vi "Puzzle 25-1.vi"() -> ()   [LabVIEW 2022 SP3]
uses:
  <vilib>/Utility/miscctls.llb/LVMapReplaceAction.ctl
  832f64d6-6221-4642-9731-2bf24a069344.vi
  <vilib>/Utility/error.llb/Trim Whitespace One-Sided.vi
  c09a35fd-dfb7-4751-8a6c-d1f927b46256.vi
  c23b235e-6b21-46d7-9deb-4925a2cb368b.vi
panel:
  in  "delimited string":string="srp: gkb zst\ngrc: pxt\nrbc: zcc mth dgq zrv\nglc: dqz zlz hqm fkn\nzpx: sfx msc hnx vjs\nmlx: tpx mfb\nfds: zqn xcf brs nmv\nfjm: qdk\nrvb: kbj\nzcj: bmc brs jtm trk\nnps: bfh ths zds\nscs: kbj dqz zfb rtp\nqrj: jsk llj\nkdj: frn tzp qrj\nrxp: mkg\nqzr: cxn hnn vhf tdd\ntkb: bvf fhp vjt\nnjz: hlq fdc\ncmj: dfp\nhmr: vbd\nnnk: bnr\nfgx: lfq gkv kms mbx\nlqr: vpc hmr dsb\nsck: kbj skd\nqhk: hgs\nncs: bnr kxr ggq mdp\nqmb: bsf zqk fhq bsz\ntjc: bsq jgq\nzzz: jtl\ntgl: fvr sbc dqz\ntht: ptz qmp qmr\nvxl: mqs tkk bfc jls mzq qpm xzr ffx\nttk: qrx\nmxz: gtz\nhrk: crj scs xbm lqj\nbcd: gdl vtg\nnrf: mqf ndq fch zvp\njss: sks zdr phr zpt\nxhd: dpc\nfkn: hhl\nkgc: gnn\ngtt: bfc jrp jdd kjp\nngh: tlh chd tkz\nfzk: gdl hhj cxk\ngtf: mmt\npgf: nzk\npxl: jdx vqx vvq\nsrc: vcn cvg xjn\nzjb: hmv rfs thn\nnfb: qzc\nsbx: txq cms kcg\nkbx: jrc bnz lpg glg\ndjg: zzz nhs vvq\nbzm: mgb frt hhf mvq\nszs: qgx khz\nkcq: bbt xkv\ntkn: frn\ncbm: mmj\nlzh: nkp nbz\njvx: cjh mhz\nnrb: kms gtf gbg trs\nhkl: kvc\nbtv: dck\nqph: vnz tbb pbh\nfdp: hhl qkx\ncmx: tjj pnh prx\ntxk: qdq vqr cjv jtv\ntxz: kqd vgr kxn\nhnz: cmj\nmsc: fdc vjr\nmgl: ljf\ntzk: srv dbg\nckg: dfd pkx\nzzx: fhq zsm cbv ndd\nvpr: lfq zcc zzr ffm\ntkk: jbk xpp hpp\ndxd: xjn rjl kpl zjg\nmkz: qfv kfq kvc\ndkb: fjm mfr zxs xtp krc\nkhz: qrx\nkhp: fgm gkb kml jkz\nsxn: tnd htx dph rxp\njdc: kmr\nkbr: zqq zgx\nchm: dcv xbj\npdr: qmp xxd zkx\nzbv: bfv dln qct\nqlj: xsm jsk rtm\nkjg: hkl pcd\ngpp: stn qxq qjh kbz\ndtk: zcm hqs fjz flj cvl zcl\nlqv: lzm\nlcx: kxd krz bnz\nlqq: qtq vks\nctp: jdc kbs svx jqq\nfpr: hls nmv\nltx: pbh vcb qgh frc blr\nmmx: qkx vpc cct\ntsp: xrc zsq\nxdt: nfs spz\nxlf: dsb qft xfh xns ngx\nrmx: xps xxn mpt prc\nnmq: gmx vxd gms src\nklf: vgj mln\nfjl: pbd hvg jvg\nvzd: jgq\nqvx: rsq\npvp: rvb hqs xxd\nchd: jlk hqm\ngpc: pgc jvb\nzdx: nmk bbt shz vdr lzq\nths: btv zdr\nrtn: qpm hbk rpt mpm\ntdt: jnq xpt\ntpd: xjb lqh\nrgf: zqj\ntzp: xhx qcm\nsjs: mdb ncp\nkrz: hlq\ncjv: rks\nvgk: bcb\ndtc: vfj zqn qbk gvn\nckh: mtf jzf\nlxq: pkx chm\ncvc: fnv zqc mrp msn\nqbk: qxq kbm\njlz: mmp chf szf pbq\nqdp: mgl npj jpm\nddm: ljt gkd bkf csg\ntdd: rsg\nrhb: brb vhm kpl\nzjg: dfp\nxbg: hkb mqf\nszd: mnz\nsbt: kzl csp jdx nhr qgk\nczq: lzg\nfmf: grv vld rjb mbk pjq\ncnm: sqp btr xrk zjb\nxdm: shz bsj skd\nsnl: lkl drt kqm qnl\nhpp: htt\nmtv: bdh jnf\nzbk: hnz rvm djg zxs\nbjp: vfj bjn bbg zns rxp\npgm: dnl clq gzt kkm\nksf: bvf qhk nzc zdh\ndbm: rnh rnm smq zcx hjn\njbd: nrb xdd qgd\npjk: ljq\nghv: nrb kqs txh gnf\ndxp: vrh rst rgg vbs\nnks: jnq jrj bmc dkc\nnqs: rsn dfm rgs vng\nkfz: ltx vck lqj zxd\ncjr: nhs mdj bkp dkj\nvcb: qmr\nqpv: kjj fbk ffh\ndcn: kbj gtz\npvd: vhf\ngrk: qrj fbz bjn\ngnl: jmk mkl\nzkj: jhh\nzxp: pmb\ngzs: ltb ffh szd\nkvt: nzk\nhrt: flj\nvmm: qnf rsn hqg nkm npb dnh\ndsv: tzk pbq vfk tcg mtn\nzxd: vhc xbj crv ngh\nbvc: mcs zms sqg fnq\nxhz: szs\nckp: zlz ttb npd\nkmr: zjk\ngcz: dkv bzb pvp rhr\npbq: btg glm khc\ncqx: vgr jzq\ntbj: ddg zlx mtk gbt\nxtx: tbc lmg qqg snf\nlsq: gkb srb\nzlj: xxz qtc hpp\nvcs: kqd dsb jbk\nnrj: mzq xlf\nffr: csg kfp tgb\nmxb: tgj\nvsg: vhz cgt qbb\nqhj: cvl sks zrt\npml: jzq zfb fmg\ndlz: fzt\nmhr: cpx svx rkx dgd\nvhj: bns ptj\ndmj: fns vkl dgr\nvvk: mnz\njjb: hmg zsq qrj\ncxk: xln\ncvg: qdk\nrqn: nxm kkm\nzpb: cvg\nxjc: ttk\ngrh: gtx\nnnj: pxb vdp jdc srd\nghf: tbb dhd kxb\nqxq: rxs\ndpn: dvh ffr znv gbd\nmnf: thd\ndzz: spm ztq vjt\ncgk: dph nbz\nrhg: zpt\nnqv: gcp pzq cmj zvt rfx\nkrq: xrc rtm\nvtg: llq lts\nnkm: kvt hck\ngzt: ngh qdq\nskn: zqn spm gpc\nfnv: hkb\nbvb: dtm dqh hhf rsm\ntxq: pkl jbb\nfrx: kkm hxb ltn\nvcm: fzk rqn jhb bsj\njtm: bql mxf lkb xtl lcj\nnnn: csm prx khj qrs rck\nqng: gzq pbh\nvhl: smt\nxxj: rlj fql mhz kms\nzxt: npk pkm zpq cgz\nhtv: htn mvf xvd qtx\nntn: qbz zjg dlg qsl\nbjz: lxt vgj ncb\ncdl: jfc\nzvt: gnl sqp\nqgk: kfp jsp\njnb: bdh bjz hxb\nrtr: dbg jhs\ntcz: tvt\nbkf: ssk qhf lkn prx\nzlc: dlz zpb bsq sqg\ngkx: rcj dck vhh xjc\nrcj: tkz\nbmc: gnn\npsg: nmt dxk jsp mcj\nqqg: zst\nvng: cqx\nrxd: dpc hpp\ntcg: vhh\njnq: pzd tmv\njxx: pxg\nxld: xns fmg fdk\nqgv: kqd zlz mfh xdm\ntct: hck gzq\nhcm: hmv rst hsr\ncsg: hkp\nvln: msq frj vcs lhx ffj\nqqv: pmp khz\nbgs: dfs gmz jdd bsj\nngd: kdh pkm tzp\nfxr: zlv zbv nhr jrj klc\nhkg: pkl qrx ktl gjs\njdh: rfh hcm qkd ghb\njfm: btv\ngjt: tss hcd zgf hdg\njzx: hck kjp xrd bxs\ntlm: smt vhf\nltn: zfq mfq\ntbc: pcq\nsrz: qhq sbc xln mvp qpm\nsdf: mrn tpx mgl gbg hcm fqk\nfxn: msc vrh bfs vvk hkp\nqfx: tbc fvx jst\nrbr: cmm zxp\nfmg: nkk kgd\ngsg: bpm lnz\nsxl: crs\nznm: qqg rfv vms qrn\nghr: htt dcv\nzrg: gbx rdr tkz\nbnd: xcm hdg fds hnz\njbk: zpr htg\nbdv: nbz ptj vlk\nlvk: htt pcd\nhmn: qzs tfc csh qbz\nqhf: scf rgg\ndzq: qls\npjq: jbl ltq gcg\nsxf: vvq tfc\nthz: mrd bgm tfq rrc thg\nbsz: brb fnr\nxhx: tdk qlr\nkdn: pld bft fqk\ntcq: lkn mgb zgz\nsfj: vlh gft lxd\nfvr: hhl\npvk: tkm bbg tqb\nmdp: lrp hdg tgb\nqkj: nzk bmj nps xhq pgf\nmxf: zkj qcm zqx\nvlx: tvt cjv zfx sct\nxhj: jsp jtz hsr rgt\nlkb: bjq vnd fjl\nlqg: xtp zqn hjn\npms: xxz hnn htr gbx\nszj: zlj fjz xzr djq chz dmj jnf\ncxs: hsr xtl\nglm: nxm jhb pcs hrt\nqjn: trb pxk\nxnx: kgd\nmfh: svq lpk\nphx: scf\nzdr: gtz\nzzl: lvv ngd jrk qhk\ncpz: bnr szd zfz dzd\ntvr: vhj nhz pxk qtz\nvhz: svq kbg gkb\nbfs: cgk nnc gcp\nfqg: ffh\nkbm: pkm\njdt: zdh dgq\nddr: npx\nkmt: hdg hls gkr vzd\nxlq: hkk tqv zjt zzf\nxxn: mmx lbt xlq\njmx: vfg qsl zqj\ngvn: bvf dzq ccx\nkzv: mpk pnv\nkht: ddg\nlxh: ddk vjs mcf gzs\ntqx: ljq kgp\nvnr: sks\nqbb: blr nkk xfp\njmz: lkq dmx dfd bhv\ndft: fcg\ndpc: hhb\nsqv: nxc\ndjl: thd rrc\nmkj: vtk tlm ggr\nvxh: kxd ghq\nkns: zcx mxv gkc lzh\nvnt: dvj\nqrp: mtf pzr\npfs: mnf cfz sbx jfm\ntlp: xrc qzs tpk psc\nkks: mzl dsf ght svl\npxq: kmt jrj sxp\nvgc: shz ddr lkq rhd\nmrn: qdk\nqls: rfs tzt\nktb: llj mzl xnv lfz\nftn: dsb\nvrs: xpt fnx mzl jxv\nzxs: rtv rdb bvg\nbsf: vht\nlrp: zpb\ngpb: ngx jnf dnl gkb\nlcg: thd vnr tht\nmgt: dbg pfp\npvv: pqb znm spz gbx rsq\npdx: dgr qng srv\ndbc: ffx xkv\nbsx: src gnn\nzhp: nnz msq gft prc\ntst: rsg rgs\nlqh: jvb\npff: lxg lbf\njqh: frx flj ftn lns mrx\nxbm: prj tsb qnf\nthd: qhq\nvck: ztv vkl dkk vdr\nmxv: kxd tpd\nvcz: mtv lnh kxz nrf\njbb: pfp\nsct: ksj xbj vhc\nlkn: tkq\nfgl: ght snj xlh\npqb: vpp tvb vgk\nbgk: ptl zfz hls mdj cfg\ntxv: pld\nltq: qhf\nfts: mfr pnx cht fhq\npgl: rrj cdd llc mtl\nzdn: hsr bsm tsp bdv vxh\nsdc: zjg csh bjn\njph: zqc xhd jnc hxb fgm\nknf: qrn ndq lxt zpt\nnfz: jgr qgh bcb\nnnz: zkx fdk hhl\njtv: xhz hhj dfs\nzsm: bnr\nbpm: vdt\npcd: vng\nvgj: nvq kht\nfck: xjc\nxsm: fjm tpd jhh\njhs: hmr\nhtn: znv jch xdd hlq zsm\nsrm: nvf tnd cfg\njqq: cbm slg\nrsg: dsb\nvqx: sqv kgc tdk zjg\nqgd: lcx mdp ssk bbg\nmgb: mlq\nxpt: hcd lrp\nkxb: zgx vtl hch\nbsm: fdc kqt\nlzq: ncf pph cxn mqf\ntsb: vhf mxz\ntrs: qsl jhh pcr\nrzf: cct vhh\nhtc: fxd llb vgs mdb\ncrt: glg tvk fhq pxt\ngvk: csp sqv rhf\npqx: qgx jmv qzk\nzqk: tzt lfs\nzhd: qkd fxh mhz\nbrb: ccx\nmth: mxg lhb cmj\ntrq: sbl frn bns\nmvp: lnz zvp\nvmb: npd\nqmr: fgm\nvzl: llc kbs fqg gnl\nzfb: nfs lxd\ndln: xdd pzr vnd\njms: xjb ccx mdj lqg pnv xjn\nvhc: kjg kcq\nffj: qvz\nqgh: lqv mfq\njcv: lfs pff zqx\ncxt: qhv cvd svl kpl\nzxc: qqv fxq djq htt dbc\nvjr: spm ghq tkn\nmht: zqx qtz xrk glk\nsgx: chm bcd rzf mhb mnf\npxp: jmk\nvld: jbx rst zns vnc\nkcd: dgr\nmlj: hnz hns rxj\nbbm: hkl lhx mqs\nnvs: rqn gtt vlh fns\ncqh: gzq\nkxt: pxb jdk gkr sxp dkc\nhbm: vxm bfh\ntgb: pbd\nhdl: kjj dmd mmj tdk jtq\njcq: vfg rtm tmf glg xjb\nqkd: dsf vxd\nnzc: grh fgl\ncpg: mmj mcf tlp\nlns: vfr slb htt cdl\nlps: cxk frx fvr msq\nfvx: fxz htr\nffn: psx bcb rhd jvz ftn phr npd\nstb: djg trs sxl lqh\nkmj: rtm pxt rhf\nqsn: vbp qxl fdc\nsrf: kgm rvm fbr thn bsx\nmdb: slb blt ddr\nggr: qnf\nlsh: jhs rvg gmz\nqfb: lkl qfq dvj\nzlz: smt\nzfx: jvq qqg xcq\nrmd: phn gfn frj\npsd: qnh vmb nrj qnf\nhml: mxt\ndbx: lvk kxn xhd vbd\nncf: kqd mtk qrd rgs\ncbv: sdc\nbph: pxl fdf jpm lpg xhx\nfmr: kxh hrg prj\nrhr: kmg kng gfn xcq xlf\nslg: qxl dqm nhz tgj rck\ngdh: znl vsr qnf\ncbn: zfq vms mrg rfv\nblr: hkk xfh\nmcs: cmm jtl nzc xgh\nmmj: lqh\ntvv: ltn cqh srp rtr\nzfz: krb\nshz: jbb ztd fch\nght: qbz csm\ndcv: nvt\nzzf: jst jdd kjp\nzmx: msn rzf rhg kcg cfz\nngz: xtz qhj lnh vgr\nxxx: vgs tvb\ncjh: zns\nsbl: dxp kmj\nrjl: tgj\ndjj: ktq ttk xxx\nqzd: fgg\nklk: jdd vgj\njrb: sqp pxq nck rkr\nzcm: mln cqx mdd\nbkk: tst rrc mmp\ngkv: mfk ssk csg\nthx: ftn sdm grl fdr\nqmm: qfb hbg qsn\nkml: bqd\nbfz: srm vht btp\nfsx: bkk zpr jmv mzq mst hxb\nncp: rhg\nncq: qfb dmd tgg\nrfx: bbg jqq\nzgz: krz gcg ghq\nthj: hmg sqg zjg mnz\nxxd: sks spz\ndxm: ndd\ncgt: vmb llb trg\nrql: mkl pxp cgk rkr\njzf: qrp pxb\ntkm: grf\npmp: qtq jfc\nvnb: frd nfb prc\nszf: frc mln qhg plt\ntfq: dgr hkb\nvks: ztd zlz gbt\nzsv: lzh tkm hgs\nkqt: tch njz nnk\nnpd: zvp\nfpx: hnn hzg qvg\nzzr: jvg gvk cgz\nsnn: bnz pkt djg mfb\nlxg: fhp\nxfp: kht\nvqr: qtc jhs szt\ntnh: ngq hjn ljt fsg\ncms: ffj kjg\nqrd: cvl\nrjr: btr cjh rlj sqv\nsfq: jdx fqg sqp ngd\nczj: sdf psg tkq qhv\ndbq: pkl vlp snf trg\nrjb: xhn sqg\nkhn: gvq gft\npxg: fqg pld\nhhb: npx\nkgm: kfp dxm\nqfv: qmp pgf\nmsb: xqq jfc dsb fvt\nmrd: vxm\nmdd: kjp\nxfg: gvq ggr zpr nkk skd mrp\nrrm: bkp vxh pvl vlk\nvfj: mbh\ngbg: cjr czq\ntkz: frj\nqfr: rfx hnz rdp nrb\ntqv: nsh gzq rdr\ngrv: lzg\nzgf: dlg hzb qlj zpq hgs\nngm: gxf szs kcq hzg\nqln: lqr jsm hmr gbl\nzcl: bcb rrc jzz\nvlt: kgd mtl\ntch: mmj rjl kjh krz qhv\nqdg: kqd lxt vxm qvz\njnx: lxd thd pdx bcd\ncrv: ggr sxb sqr\nhsr: tmf zjk\nfmj: scg dft lxg rxp\nnpb: kcq msq tsv\nsdm: mrd\ndfp: mmt gtx\nktl: jth gdl slb skx\nddb: trk csp mgl lzj\njzr: ckh dph brs kmr\nmnt: srp xtf gqz\nzqc: xvf srb\ntpk: rdb\ntmn: kbg kjg jxk chd\npnh: qjn tpx lpg\njnf: kbg ttb\nthg: mxt zjt vsr\ndnh: xft gbt\ndbg: flj\nzbn: hlq tlp zhd xjn\nbzb: qdq dpc\nmmp: mkk vhl\nmbm: znl\ntxh: dvj\nfpd: jbx zxp qpv\nrdt: ptl jrk fzx\ngpj: mrn\nrzj: kbg tsv lpk\nvhh: vpc jth\nsqg: tpd mcj\nhlf: dck tcg sck fsv jss lfr\nzcx: mxg xkn jsk\nxnv: xcm xkn\nnvq: ktq\nrzz: lvh sqp dtm hbg\nprx: xjb\nsxg: rbr sxl pbd\nvlp: gfx gft\nltc: bql pzr gvn\nhck: htg\nqtk: nbb mbm mkk\nksj: tvt\njbn: qzd ffh lkl\nnhv: fql kdn\ndzk: hqm lsq xbj rxd fnv\nkgn: gfq ltb pvk jbx zlf\nlsv: qrc rtp kxz chm tlh\njsm: hcj bzb mbm\ntbb: bbm nvq\ntgq: cmm vnt grf xpt\ncvv: mvf xnv gnl ngn\njmn: tdk rzn rxs cbv\nhbk: fxz\ndkv: srb mdd slb\nzlf: dvj\nnkj: sbl svr pxb krb\npgc: kmj\nrqg: grl nlj hzr tsv vhl hhj\ndkk: gqz qft vlh\nzzs: hjp bvm pgc ggq vvk\nqfm: tfc tsp smq mfb\nmvq: gfq mlq\nfrd: fch dfk\npsx: mrg djl dmx prj\nbvg: gtf tzt kxd mxb\nbfc: phn\nfxx: hgs qbt knc qrp\ndqm: vxd zsr\njhm: zdr gbr ckp fkn nrj kgq\nxjq: htx khj\nchz: nxm svq szt\nsjt: pnv\nvfg: vht kzk hls\npqd: gjs vdt zlx blt\nrcs: pnx hnt jpd qff\nsvr: tgj\nvqc: qfq\nnbb: bdh ncb\nktv: trb vzd\npph: pbh cct\nlkd: lbt lsh zcm xxd\njrp: njh dcn qhq\njbx: rjb\nmpm: qnh ncp qrd pml\nbsq: qbp\nbdp: vzd kxr bhj mtf kjh\nqft: ztv\nfxz: xpj qrx\nfrn: dxm\njrt: xrk bsz rfh\nrhd: xpp jlr mxq\nfvb: gtx rkb tcq hbx\ndrt: gkc mhf\nfnq: jnq xlh vsm lvh\nffl: khj\njvb: qxl\ntlf: rrc dfk gxf bcb\nvbg: tlm hhb vpc fmr\nmbh: cmm\ntgg: dvh\ntgx: qhk mvq fcg dxd cvg\nrtp: jvq cxn\nzxb: zkv tvb vdt gbx zkx\nvtl: llq qzk rcj\nvdc: xrb\nbbs: rjl\nxsg: jnq gkr mdj jzf\nkqs: nck qkl vss sxl\nzdh: dsf\njlm: lzj mcf qcm zkh\nzkn: xkv xfp qzc klk\nkmg: rvg kcq\nfxc: rdp cnr zxs kzk jch rgg scf vcn\njxc: spf hbk\nbgb: nmt qrs cmm svr\nnlj: hzg ncb\nngn: rfs crs\nbjx: ztd kvc\nrkn: fqg bzc kbm dmd\njsk: tjc\nktq: chf\nxrk: tkb\nlld: lqv mnf\ndnq: hvt krb cpx lkn qnz\nttn: qnl cxs tdt llj sxl\npng: sdm ghr mtk\nhjn: bsq\nsmq: qcm ngn\nvnc: bsf dgq shm\nlfq: dqm qbz\nvgs: gqz\nxnf: hdg kjj mfk jdc\nzms: crt fbf qdp tmv\npvn: mfk svx zns htx fbz\nnkf: rsn fck gpb pcd\nksn: csh bfv phx\nvhm: mqv dxm bql\ntfc: mxg hzb\ntnp: ffj lld\nrhf: qfq\ntxj: srb vsr btg rvb fns\nkzp: jrt qhv nzx tqx\nngq: pzq bnr mht\nnbf: cbv sxp jrc hjp\nkhq: sqf pgl rtv dxm\nmtq: zqx kbz frt nck\njzq: frj\njhb: xpj qtc vhl\ngqx: mqs zfq qnk\njkx: bfz pvl gkd frn\nqnz: vxd qzs\nhns: qzs zlf\nzds: qkx xfp\nhjp: jrh nnc\nqst: qzk kbb mnt smn\nvfk: sqr xqh qzr\nvpp: xld hkk kcd hkb\nmkl: zqn\nbpk: hzk llq xns kht\nmvf: pxg\nkbz: zlf cfg stn\nxgc: gcp jzf vbp gmx\njks: ztd znl rfv\nxdq: mlj ksn nxc ljf kqm pvl\nmcf: frn\ngbb: sbt fzx zsr plf\nlfs: jnq kdx\njhc: llc vvl mbh qkd\nptl: pxz csm\njtq: ddx\ngzv: cms ncp cxn\nprj: bfh\nrrc: jzq\nkxr: rvh hzb csm\nvbv: vdc jkx rkx tkm\nxft: ttb\nddg: bdh\nxcm: jrh dlg\nhdc: jgq cxs bsx pzr\ndkh: zhd kdj jpm jvg\nggn: ttk cqh jth\npkt: zvc khj bhj\nnhs: ghq\nrdq: jzz vnr zrt\ncvd: llf kqm rck qfq\nzsc: jpd pmb nhv scj htn\ndgd: cxs bjq qpv\ngbd: bvm mxb jdt\nvdp: jgp dvn rzn\njkz: kfq npx\nzjt: qvg qrn\ndrd: rst hns jrk mrn\ndtg: bbj gkr rjh\nztq: jvb pxz nhz\nxln: gbr\ndgq: svl\nzfg: gtf mvf ddx sqp\nlkk: kxh pvd ljr gzt vnr\nmhf: ghq mlq\nhqr: scg rxj qkl tkq\nmgm: ptj pbd rxp rtv\nlzj: xcf lfz\njtz: jpm snj krb\nsfg: xng dvn fdm kbf\nqff: csp pxz\njxk: mkk qnh mbm\nxpj: jzz\npcs: ztv lnz\njrk: xkn rkx\ndzd: krq tfv xth\npsr: rlq fsv rks gzv\nfrc: nfs\ntjj: sfm\nzkh: bsq rxs\nfjz: srp\nkxz: cxn jqv\nscp: cpg tgq ptb qzd\nxtp: qbp\npns: hhb cdl\ndzj: cgz gpj lkn gkc\nfvc: rrc hqm ngc xjc\njhh: bvm\nplf: xgh sxg nhs\nllf: ffl xth hdg\nbjq: ddk gms\ncrj: ngm ngc vlt\nqhv: jtr\nvss: pmb pxn bjn tfc svr\njnt: fcg jxv tpk kbf\nlrh: chd kbr hqs ztv\nhzb: txh jrc\nrkx: nnk\nxns: kgq lhx\nkcn: kkm zrt lqj xbv\nxrb: mmt zsr mdj\ntqb: bds mkg kdx\nblt: lzm\nxbt: skn dzq kgm qlr\nrvh: shm jxv\ntrg: btv\nmrx: tsv mfq\nxtf: zpr vtk\nzqq: rzj vbd\nxrc: mpk brb\nbkj: pff zbv mgb crt jbn\njvg: fpr gnl scg\nlbf: xpt\nxzr: znl\npjn: trg qft pvd pgf xft\nccx: mhz ffh\nnvf: kms\nlkq: zqq\nbtg: lxt spz\nrlj: kmr kqm\njqg: mkz chg xkv ncj\nxth: vcn\nbhj: vht bsx\nxvd: ggq qgd trb\njgp: ltc tzt mkl khj\ncqt: gkd gpj qht krn\ngmx: qsl zxp\ngjs: ksj mtl\nqtc: qzc\nhvl: gcg gkr fnr nrb\nfxh: nkp svx\nrxj: pkv gfq\nfnx: lvh kgp\nmhb: mkj nsh qpm xqq\nchg: pfz rqr lqq qft rsn\nbtp: rgg vnt kgc dkc\nrzr: vrv nkj grk bds\njpd: vvl mgm\npkv: xth bbs rrj ggq\nkdh: gms gnl\ntpq: mvp qnh kxn\nkrc: mxg bnr ffl\nvnd: hmg\nzlv: mfr bft dzz\nnfg: jlr ksj nvq lnh\nrld: lxt svq hch\nspf: ptz nfb htc\nvdt: rhg sxd xtf\nhvt: trk rnh bnz\nlfr: qvg tst xft tcz\njtg: jbd lqg hcm rvm\ncdd: brs kdx npk\nhqg: gmz xhd frd\nbgm: qvz vnz\ngfn: bxs\ncrs: fql\nvcr: xcf pxn jsp shm\nvjs: lzg jtl\nlfz: kjj tjj\nfdq: pqz qbp qcm\nlnh: zfq\nnmk: kxn xtc phn\nnpj: lkl mlq mfk\ntcc: tss nhz szd kns qzs\nlts: jfc sbc\njbl: ndd\nkgd: jmv\nsnf: vms\nlmq: xxx bpm djl vng\nkbs: gpc\nphn: kgq xfh\nkzn: thz blt mxq sct hml\ndts: hvt bql ggq\nvvl: zzz ktv ksf ght\nllb: gqz\nvlk: jdc mnz\nljr: ggn vnr nvq\nfdk: bbt\nnkk: snf\nqbh: krz tdt cvd rhf\nhxq: jmx vdc dvh cbm\nrll: rdr mst jnf vgk sbc prj\nhzr: tbj jjm xqq\nzrv: lrp grh txh\nqtx: jcv stn tkn\nlph: rjh nmt crs kgp\nkxd: rhf\ntvk: pfd pjk\ndhz: gbr gfn fdp kbr\njrh: scf\nngc: gss hnn xnx\nzqn: rtm ktv\nqgx: nvt\ngrd: rrj bsz qjn lzh\npfz: ncf tnp qdq\ntzt: zkh\nzhh: thx mst tsb xhz\nxqh: tct bxs kml vmb xzr xbv\nxpp: xfh nzk\nlzm: mxz\nbtr: jtr krb\nzmt: jfm zxq fmg chf dgr\nmcj: nmt vcn vjt\nkcg: szt jbk\nqjh: pvl drt ktb\njls: tlf pns\nnbz: vjt\ngcg: txv fnx\ndfn: kkh rsq kmg jnb\ntss: nlh xmq kzv\nlbd: jmv gqt nkm ngm\nrfh: trk\npzq: svl hcd\nfdr: vsr blr ngx nlj\nljt: zsq tmf\nxlh: txh rhf\ntlh: nbb xjc\nfhh: fck qvz lcg ggr zrg mrg zrt\nhsp: vnd czq pbd lzg\nvsp: jhh fqk jtj bsm qff\nrnm: ffm jtq drd tgg\ncnn: mbh qnz kbm jrc\nptj: jdk\nxng: nhr jnt pnv\ndqh: mvq qgd dlz\nhbg: grh tjc nnk\nvbp: trk vbs\nrsm: glk ffh ljq\nlpc: vcz jgr lxq\nszt: mln lts\nnmf: ddx bvf zsv sxf\nnxm: gqt\ntcn: dbg gbt lmg dfk\ngqz: tvt bqd\nfbr: zsr fpr qct\ngrl: kgg ggn\njst: kht\nmxt: frj\njqv: mtv gtz jvq\nqhg: npx\ngdl: gsg\nvlg: jjm xsq tbj vgk\nsrd: vqc\nznv: fcg vcn\nhnn: kht ptz\nlpg: gmx pkm\nrdp: zvt tpd\nxtc: ftn kbb jlr zgx\ncfz: lqv pkx kml\nxtk: xdt lcb qpz txq pfp\nhhl: lpk\nbkh: bqd ckg rkv jkz\njlr: gss\npqz: pdq qhf jdt\nlrm: skx tsb hbm sfj bhv\nsbd: ncq fhq zsm pxn pxk\nxcq: xbv qpz\nvcx: htg bbt tlf gzq jfm\nnlr: ddg dfk ncf kcd\ndbn: dlz mqv qrj nhv\nzkv: hkp kzl\nnsh: rks pph\ndfs: jzz pns gss\ncgs: ssk zpq dtg rgt\ntdg: zdr qkx psr qtk\npfd: zqn mdj\nrvv: sqf xdd jtz snj\nrtv: czq llc\njvz: nzr qgx qfx fkn\nclq: bgm tpq bxs tdd\nfzt: hjn rfh\nmrg: sxd bjx klf\nfmx: pjk pxp svr rgf\nkbb: mdd sjs\nlqm: kvt rks qvx\ntfm: bjp mnz shm dxk\nnlh: rdb bmc\njjm: gfx mnx lqq\ncpx: pcr mmt\nzlx: dbg\nqnl: kbz sfx lcj\nccp: rrj jtr rvh tkm\npxb: bbs\nkvm: skd fgm txz\ncsb: mlx sfx cbm gcp\nrnr: zvp fvz kng vkl tcg qtq\nfbk: jxx xpt bnr\nfxq: pcs bjz vfr\nkdk: qtz jxv vvk\nnnc: rfs\nlbt: gqt hbk\nfsv: mrd cqx\ngqt: kgd\nvnz: hkl rsn\npcq: dsb khz qpz\nhgs: pzq kzl fgg\nkpl: tpk mkg qbp\nddk: ffl\ncbc: jsh lcj dxm tfv\nvfr: xsq txq\nxsq: ttb\nhch: kgq smt\nmhg: nfs bzb xsq tcz dcn\nhmv: rst jxv\nbbg: bbs txv xcf\nzvm: zcx kgc trq htx\nlcb: mvp frc kcd rxd\nnck: qzd bsf\nngx: mtv\nkvc: llb\ngfx: fch ncb\nzlr: sxf qrs psc kjh vqc\ndlg: rgf\nqzk: jlr\nbzc: tjj nvf hcd sjt\nhfp: sjt dxk qxl zpb\nlvv: fnr nnn bsf\nsqr: tct skx\nmtf: njz\nmst: xpj\nlcz: rrj jxx dft jqq\njgr: gvq hkl\nxrd: fvx zkx sxd lkf mfq vbd\nvsm: sfm bmc\nmrp: mtk ghr\ngfz: ths tzk jfc txk\njtj: rrj hnx cln\nxxt: hnx xdd rgt lfq\ngxf: cct\nsrv: cdl mqf\nfdm: ddk rxs pcr\nccf: rld lhx rdr xlq rtr\ncgv: hzk png vnb phn\nhnt: qrs fdq glg\ncht: ddk cmx\nqrr: mbx phx bft hjp\nhtg: fdk\nfbf: jbl hdg vvq\nqnk: ths bjz jls smn\ntqs: zqc rgs vlp lld xxn\nkxh: qgh bpm rkv\nmpk: mhf rgt\nzsd: stn pzd qdk sjt\nmtn: hbm vng\nhmg: kfp\ngmn: zds mfh gbt chf brc\nvgr: qgx\nblm: vgj ctb rtr lpc\nskr: vrh tfz rgf xtp\nphr: mrx nvt\nknc: nnc tlp bzc\nqlg: kgg zpj pqx lqm rfv\nqbt: jxx rhb qxq\nxnk: lhx hbk dcn xtf\njsh: grv gfq pfd\ncln: gpj zns vbp\nnjh: mst mxq\nmbk: qjn kdk ltb\ndjq: vtg dnh\nplt: snf lxq hbm\nncn: mkg tfz ztq\nbmj: lkq vtg rxd\nqsh: vsg qlg pdr xvf\ntvb: pvd\nqkx: tgl\nlqj: fns\nqtz: fjm grc nmv kqm jch\ncfg: dvh sfm\ndhd: sxd vdr rfv\nkgg: lxt\ndlh: fvr vlt vtk tcz\nzpj: lnz bbt xbg\ntnd: gnn\nlcj: tfz\njfn: rsq dfk jks rmd\nzxq: mtn lpk hml\nsft: npk zfz qsn jrh\nvff: dlz qct krq pxk jtl\nqpq: qng qmr rgv ncp\njlk: zgx qtq hzg\ndvn: grv xsm\nmsn: fck xxz\nrzn: zqk mxv\nplq: mxt sjs bqd dck jbb\ntzs: lxd mtk xsq rvb\nhzk: pkx\nthn: nvf pjk pdq psc jxv srd jvx\nnhr: tgg rck\nmtm: pfp qrd hhj fns\nskx: kjp\nfrt: fzx grc lzj\nmbx: csh kms\nhvg: qct srd qgk\nhnx: gkc dsf\nbds: bhj dzd\npzd: jmk csh\nndq: gxf xnx\nkfq: xjc\nrnh: zpq xjq\npkl: ztv\nprc: mqs\nsxb: gbr vcb ddr hkk\nrlq: gvq qvg\nnzx: kjh dxp jjb kbm\njvq: zst\nfss: zst nfz znl nsh\nhbx: vfj mlx gtx\nbns: xjb pld\nmfb: lbf\ngzk: qlr rdt fbz kdh\nrqr: zrt hrt xln\nmpt: vdr rlq smn lqv dbc\nbrs: src\nsqf: jvx pxt dkc ksn\nrjh: llj vqc ltq ghb\ngkd: lbf\nxmq: sjt ncn pxt\ntfv: bft dfp\nsfm: spm zjk\nghb: zqj\nxxz: pfp\nffx: lsq tlm\nfqk: jch\ncnr: pxn tnd scg\njnc: qhq qhg gfx cvl\nddx: dph\nnxc: fgg nkp\nzcc: vcr btr\nmxg: zjk\nlfp: rnh gpp bsf psg\nqtp: nvs bfc jxc zlx\nkqv: xjq jtq fxh txv\ntkq: zkv\nscj: zqk cjh cht\nmqv: phx pfd\nctb: fch lqr djj\nmfr: zxp vxd\nbsj: lzm htr\ndtm: mxb grf tkn\nfnr: grc pcr\nsfx: ljf fgg\nvbs: vqc tmf\nkrn: fhp vsm mlx\nxbv: qvx\nptb: vzf nlh pdq ljq\nkbf: dkj fhp\ngkr: rdb\nqrc: ckg msq qvx\nhqs: hck hzk fpx qmp\nqrn: vxm ktq\nkhc: pns ktq qmp\nlmg: lqv xtz\nkfn: shm qxq qkd xtl\npxn: mzl\nsfr: ndd zkj hbg qhv\nhtr: jdd\nvjl: kfq jph mxk khn\nbfh: jth\ngmz: xnx qpz\ngkk: jdk qhf ljf bvm vrh\nkld: bjx qzc kgg rkv\ndkc: bfv\nxlm: pdq tgb fzt zxp\nfvz: smn qhg fzk fjz cqh\nrpt: phr qmp mqs\nntm: tvk mlq rvm ltq pld\nrrj: sxp jgq hkp\nxps: qtq vhh ndq\nfdf: hmg pgc tpx kzk\nbbj: psg dft nkp\nkkh: mzq xqq rsg ksj bqd\ndfm: blm mxk sck pdr\nnzm: gcp pjq qbk zqx bfv\nmxk: mgt qph vcb\nptz: gdh\nffm: kdx\ndkj: rlj glk\nlrz: zlj znl zmt kvm\nvlh: zpt mln\nrvg: hch\nbkp: jdk kgp\nfzx: kzv\ndxk: nhz\nbnp: btv kbb tdd ghf\nmnx: vms gss vng\nghq: rtm\nfsg: svx dlz kbs\nfxd: mxz nvt klk dmx\ngrf: nmv\nklc: grf qkl zqj\nlkf: dmx scf vpc tht qqv\nzvc: ckh dzq jsh\nvnx: vzf jbl pzq kzl\nrkb: dts qlr lvh tqx kdx\nxgh: ggq pmb\nmkk: mqs\nvpv: zsq ght cjr qkl\ngnf: phx zzz xkn jtr\ntnr: gqx hml qfv vks\njdx: jrj mvf sqv\nccz: khn msb ksj lnh\nkzk: pzr\nxcj: cbv vhj bvb rkr\nrkr: npk\nljl: qsl glk trb vnt\ncxf: bjz nfb njh cjv vgs jxc\nhvs: fpd jsk mvq rhb\nvrv: dmd nnk qmb ffm qls qmm\nqzc: mtl\nxtl: pxz\ntfz: hhf jgq\nxvf: vbd tkz\nfbz: vvq\ngms: fql\nxhq: qtp nlr xbg nrf\nbhv: gsg xns\nnvc: hlf qph mrm sct\njmk: hhf\nvzf: snj pxp\nvkl: mgt rdq\nbrc: pmp sbc mxq\npnx: mgl hnz\ncgz: qsl\ndnl: jst dcv hch\nxhn: ltb svl hdg\nncj: tkk kvt lvk\nhzj: vdc ddx vnd pzd\nhcj: dqz rkv cxk\nqht: lxg psc kbf\ndfd: thd lpk\nkng: chg tbc\nhrg: xtz btv hrt vgs\nnzr: zgx xtz vtk\ntmv: rbr fqg pzd\nlhb: ghb lzg zkj zdh qbz\nfvt: klk sdm tnp fdp\ngbl: xhz fnv rvg\nrgv: fxz tfq bsj fpx\nmrm: llq klf qvx xdt\nsrb: rcj"
  out "Set 2":set{string}(c389)
  out "nodes":set{string}(c389)
  out "Map":map{string, set{string}}(c390)
  out "String":string
  out "Set":set{set{string}}(c389)
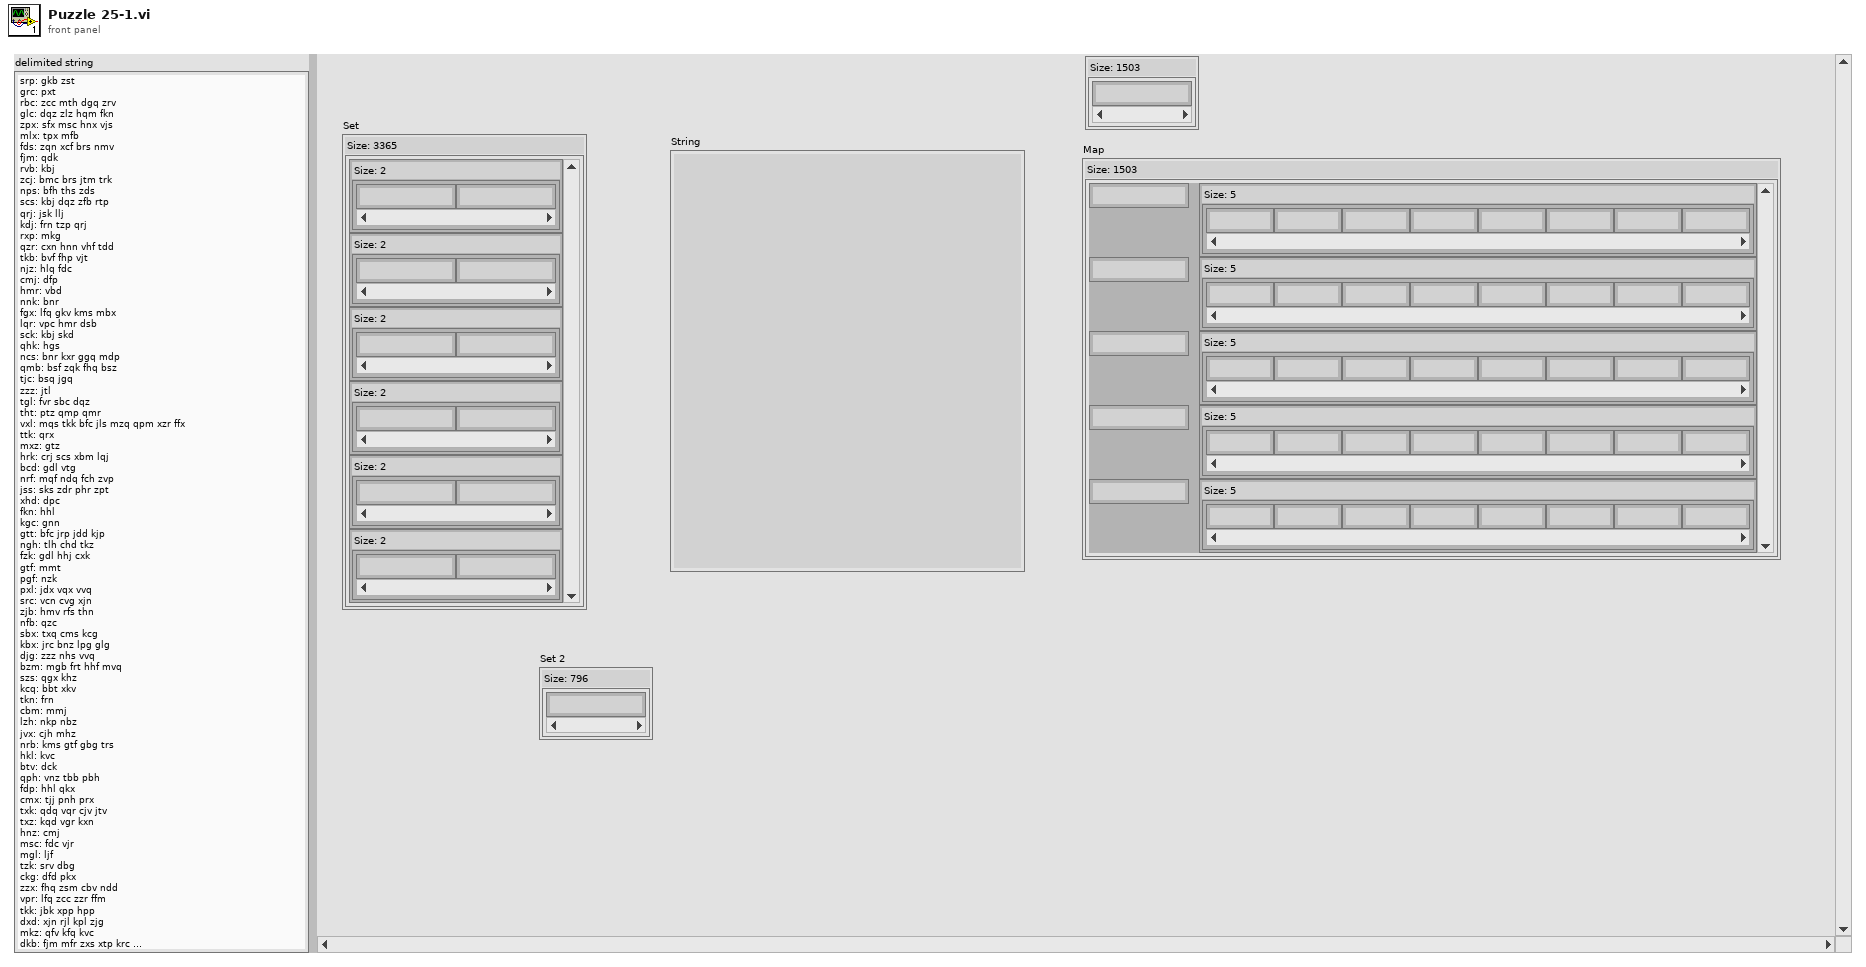
[diagram p1: front panel]
types:
  T1 = typedef "LVMapReplaceAction.ctl" = enum32{"Modify Entry only if found", "Add or Modify Entry", "Delete Entry"}
  T2 = enum16{"open", "replace", "create", "open or create", "replace or create", "replace or create with confirmation"}
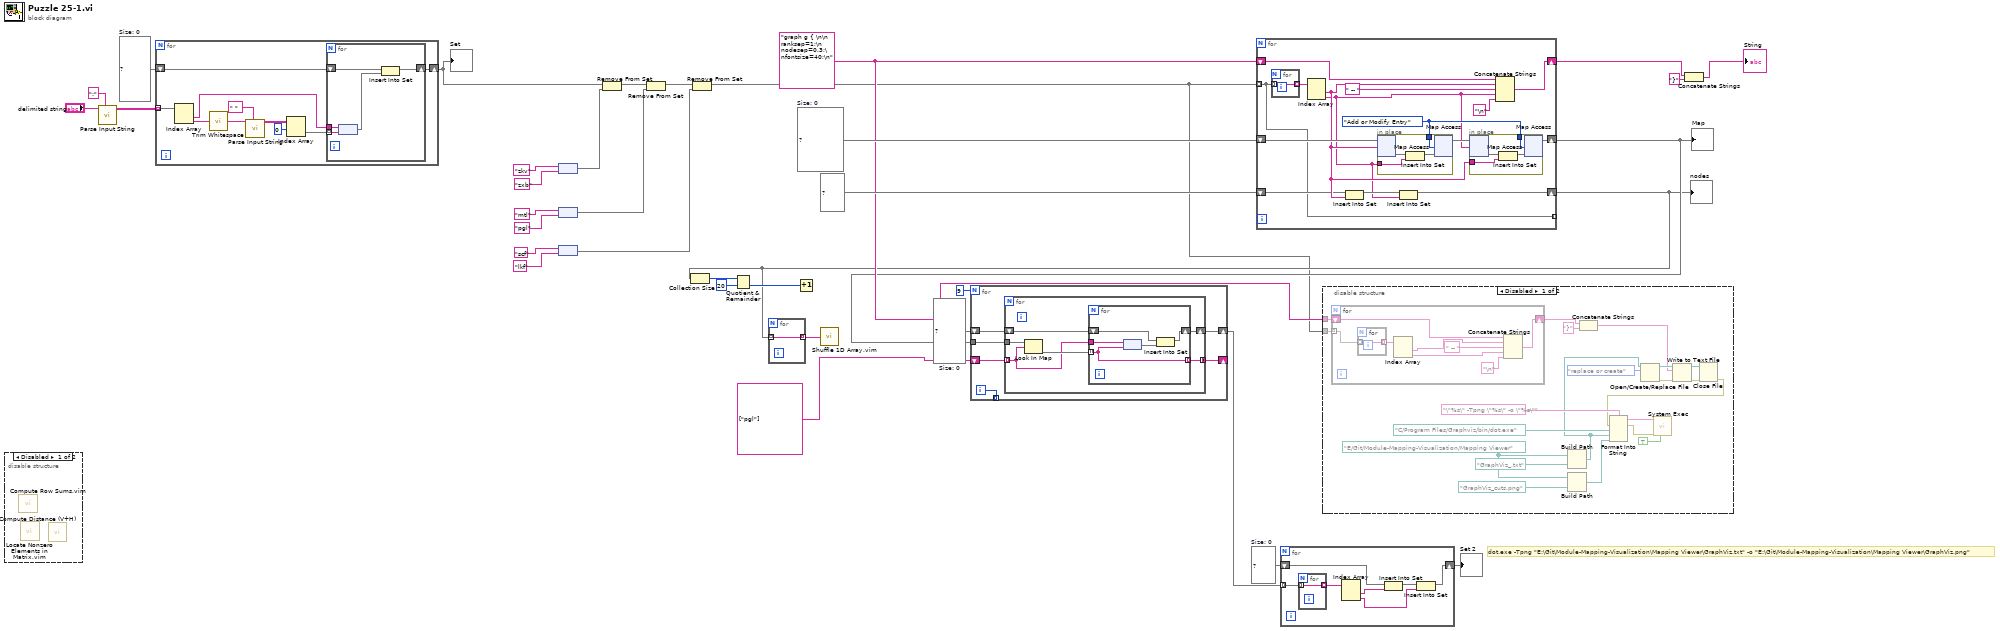
[diagram p0: block diagram]
diagram:
  w2 = set{string} {}  # Size: 0
  w18 = set{set{string}} {}  # Size: 0
  w24 = "graph g { \n\n    ranksep=1;\n    nodesep=0.3;\nfontsize=40;\n"
  w31 = map{string, set{string}} {}  # Size: 0
  w32 = set{set{string}} {}  # Size: 0
  # "dot.exe -Tpng \"E:\\Git\\Module-Mapping-Visualization\\Mapping Viewer\\GraphViz.txt\" -o \"E:\\Git\\Module-Mapping-Visualization\\Mapping Viewer\\GraphViz.png\""
  n1 = disable-structure shown="Disabled" {
    frame Disabled {
      n2 = call "Compute Row Sums.vim"() -> ()  [unwired: 11 in, 1 out]
      n3 = call "Locate Nonzero Elements in Matrix.vim"() -> ()  [unwired: 11 in, 1 out]
      n4 = call "Compute Distance (V+H).vi"() -> ()  [unwired: 11 in, 1 out]
    }
    frame Enabled {
    }
  }
  n5 = call "Parse Input String.vi"("delimiter (Tab)"=":", "delimited string"="delimited string") -> ("parsed string"=w33:string[][])  [unwired: 9 in]
  n6 = for {
    tunnel: w33 -> [w45] mode=indexing
    shift-right: [w38] -> w16
    shift-left: w32 -> [w37]
    n7 = Index Array(array=w45) -> (element #1=w39:string, element #2=w44:string)  [unwired: 2 in]
    n8 = call <vilib>:"Trim Whitespace.vi"("string"=w44) -> ("trimmed string"=w36:string)  [unwired: 1 in]
    n9 = call "Parse Input String.vi"("delimiter (Tab)"=" ", "delimited string"=w36) -> ("parsed string"=w42:string[][])  [unwired: 9 in]
    n10 = Index Array(array=w42, index (row)=0) -> (element=w40:string[])  [unwired: 1 in]
    n11 = for {
      tunnel: w40 -> [w49] mode=indexing
      tunnel: w39 -> [w50]
      shift-right: [w47] -> w38
      shift-left: w37 -> [w46]
      n12 = node(w50, w49) -> (w48:set{string})
      n13 = Insert Into Set(10:w48, 11:w46) -> (3:w47:set{set{string}})  [unwired: 1 out]
    }
  }
  "Set" <- w16
  n14 = node("zkv" ("element"), "zxb" ("element")) -> (w4:set{string})
  n15 = node("mtl" ("element"), "pgl" ("element")) -> (w12:set{string})
  n16 = node("scf" ("element"), "lkf" ("element")) -> (w8:set{string})
  n17 = Remove From Set(10:w4, 11:w16) -> (3:w13:set{set{string}})  [unwired: 1 out]
  n18 = Remove From Set(10:w12, 11:w13) -> (3:w11:set{set{string}})  [unwired: 1 out]
  n19 = Remove From Set(10:w8, 11:w11) -> (3:w7:set{set{string}})  [unwired: 1 out]
  n20 = for {
    tunnel: w7 -> [w51] mode=indexing
    shift-right: [w62] -> w27
    shift-left: w24 -> [w61]
    shift-right: [w58] -> w22
    shift-left: w31 -> [w60]
    shift-right: [w52] -> w21
    shift-left: set{string} {} ("set in") -> [w53]
    tunnel: [w51] -> _ mode=indexing
    w57 = LVMapReplaceAction."Add or Modify Entry" ("action")
    n21 = for {
      tunnel: w51 -> [w70] mode=indexing
      tunnel: [w70] -> w65 mode=indexing
    }
    n22 = Index Array(array=w65) -> (element #1=w56:string, element #2=w54:string)  [unwired: 2 in]
    n23 = Insert Into Set(10:w56, 11:w53) -> (3:w55:set{string})  [unwired: 1 out]
    n24 = in-place {
      in-place-border: w54 -> [w69]
      in-place-border: w57 -> [w66]
      n25 = in-place-map #1(w60, w56) -> (w68:set{string})  [unwired: 1 in, 1 out]
      n26 = Insert Into Set(10:w69, 11:w68) -> (3:w67:set{string})  [unwired: 1 out]
      n27 = in-place-map #1(w67, w66) -> (w59:map{string, set{string}})  [unwired: 2 out]
    }
    n28 = Insert Into Set(10:w54, 11:w55) -> (3:w52:set{string})  [unwired: 1 out]
    n29 = in-place {
      in-place-border: w56 -> [w72]
      in-place-border: w57 -> [w71]
      n30 = in-place-map #2(w59, w54) -> (w74:set{string})  [unwired: 1 in, 1 out]
      n31 = Insert Into Set(10:w72, 11:w74) -> (3:w73:set{string})  [unwired: 1 out]
      n32 = in-place-map #2(w73, w71) -> (w58:map{string, set{string}})  [unwired: 2 out]
    }
    n33 = Concatenate Strings(w61, w56, " -- " ("string"), w54, "\n" ("string")) -> (w62:string)
  }
  "Map" <- w22
  "nodes" <- w21
  n34 = Collection Size(1:w21) -> (0:w28:i32)
  n35 = Quotient & Remainder(x=w28, y=20) -> (floor(x/y)=w23:i32)  [unwired: 1 out]
  n36 = for {
    tunnel: w21 -> [w75] mode=indexing
    tunnel: [w75] -> w29 mode=indexing
  }
  n37 = Increment(x=w23) -> ()  [unwired: 1 out]
  n38 = call "Shuffle 1D Array.vim"("array"=w29) -> ()  [unwired: 4 in, 1 out]
  n39 = for {
    N: 9 -> [_]
    tunnel: w22 -> [w81]
    shift-right: [w79] -> _
    shift-left: string[] ["pgl"] -> [w80]
    shift-right: [w78] -> w3
    shift-left: w18 -> [w77]
    tunnel: [w76] -> _ mode=indexing
    i -> [w76]
    n40 = for {
      tunnel: w81 -> [w87]
      tunnel: w80 -> [w85] mode=indexing
      tunnel: [w84] -> w79 mode=concatenating
      shift-right: [w82] -> w78
      shift-left: w77 -> [w83]
      n41 = Look In Map(map=w87, key=w85) -> (value=w86:set{string})  [unwired: 1 in, 1 out]
      n42 = for {
        tunnel: w86 -> [w91] mode=indexing
        tunnel: w85 -> [w92]
        tunnel: [w91] -> w84 mode=indexing
        shift-right: [w88] -> w82
        shift-left: w83 -> [w89]
        n43 = node(w92, w91) -> (w90:set{string})
        n44 = Insert Into Set(10:w90, 11:w89) -> (3:w88:set{set{string}})  [unwired: 1 out]
      }
    }
  }
  n45 = for {
    tunnel: w3 -> [w99] mode=indexing
    shift-right: [w94] -> w1
    shift-left: w2 -> [w93]
    n46 = for {
      tunnel: w99 -> [w100] mode=indexing
      tunnel: [w100] -> w98 mode=indexing
    }
    n47 = Index Array(array=w98) -> (element #1=w97:string, element #2=w95:string)  [unwired: 2 in]
    n48 = Insert Into Set(10:w97, 11:w93) -> (3:w96:set{string})  [unwired: 1 out]
    n49 = Insert Into Set(10:w95, 11:w96) -> (3:w94:set{string})  [unwired: 1 out]
  }
  "Set 2" <- w1
  n50 = disable-structure shown="Disabled" {
    disable-tunnel: w24 -> [w121 _]
    disable-tunnel: w7 -> [w101 _]
    frame Disabled {
      w115 = path "E:/Git/Module-Mapping-Visualization/Mapping Viewer"
      n51 = for {
        shift-right: [w127] -> w102
        shift-left: w121 -> [w126]
        tunnel: w101 -> [w124] mode=indexing
        n52 = for {
          tunnel: w124 -> [w130] mode=indexing
          tunnel: [w130] -> w125 mode=indexing
        }
        n53 = Index Array(array=w125) -> (element #1=w123:string, element #2=w122:string)  [unwired: 2 in]
        n54 = Concatenate Strings(w126, w123, " -- " ("string"), w122, "\n" ("string")) -> (w127:string)
      }
      n55 = Build Path(base path=w115, name or relative path=path "GraphViz_.txt") -> (appended path=w106:path)
      n56 = Build Path(base path=w115, name or relative path=path "GraphViz_cuts.png") -> (appended path=w118:path)
      n57 = Concatenate Strings(w102, "}" ("string")) -> (w105:string)
      n58 = Open/Create/Replace File(file path (use dialog)=w106, operation (0:open)=T2."replace or create") -> (refnum out=w108:refnum<file>, error out=w109:errorcluster)  [unwired: 4 in, 1 out]
      n59 = Write to Text File(file (use dialog)=w108, text=w105, error in=w109) -> (refnum out=w111:refnum<file>, error out=w110:errorcluster)  [unwired: 1 in, 1 out]
      n60 = Close File(refnum=w111, error in=w110) -> (error out=w104:errorcluster)  [unwired: 1 out]
      n61 = Format Into String(format string="\"%s\" -Tpng \"%s\" -o \"%s\"", error in=w104, path "C:/Program Files/Graphviz/bin/dot.exe", w106, w118) -> (resulting string=w119:string, error out=w103:errorcluster)  [unwired: 1 in]
      n62 = call <vilib>:"System Exec.vi"("run minimized? (F)"=TRUE, "error in (no error)"=w103, "command line"=w119) -> ()  [unwired: 5 in, 4 out]
    }
    frame Enabled {
    }
  }
  n63 = Concatenate Strings(w27, "}" ("string")) -> (→"String":string)
